vi "[P] Upload To Server.vi"() -> ()   [LabVIEW 2014]
uses:
  Sensor Reading.ctl
  Enum.ServerUploadState.ctl
  <vilib>/regexp/Match Regular Expression.xnode
panel:
  in  "Timeout":u16
  in  "Control Port":u16
  in  "Fail Silently?":bool
  in  "Data Port":u16
  in  "Server Address":string
  in  "Message Q":refnum<queue>
  in  "Data Q":refnum<queue>
  in  "Sensor Reading":T1
  # "INPUT PARAMETERS"
  # "INTERNAL VARIABLES - could possibly be set programatically..."
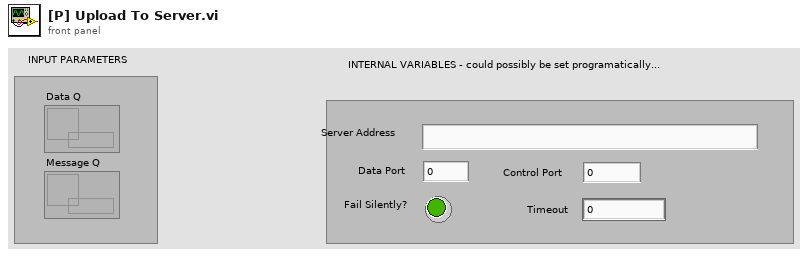
[diagram p1: front panel]
types:
  T1 = typedef "Sensor Reading.ctl" = cluster{"Sensor Name":string, "Timestamp":string, "Data Chunk":string}
  T2 = enum16{"Standard", "Buffered", "CRLF", "Immediate"}
  T3 = typedef "Enum.ServerUploadState.ctl" = enum16{"NotConnected", "Connected", "Error"}
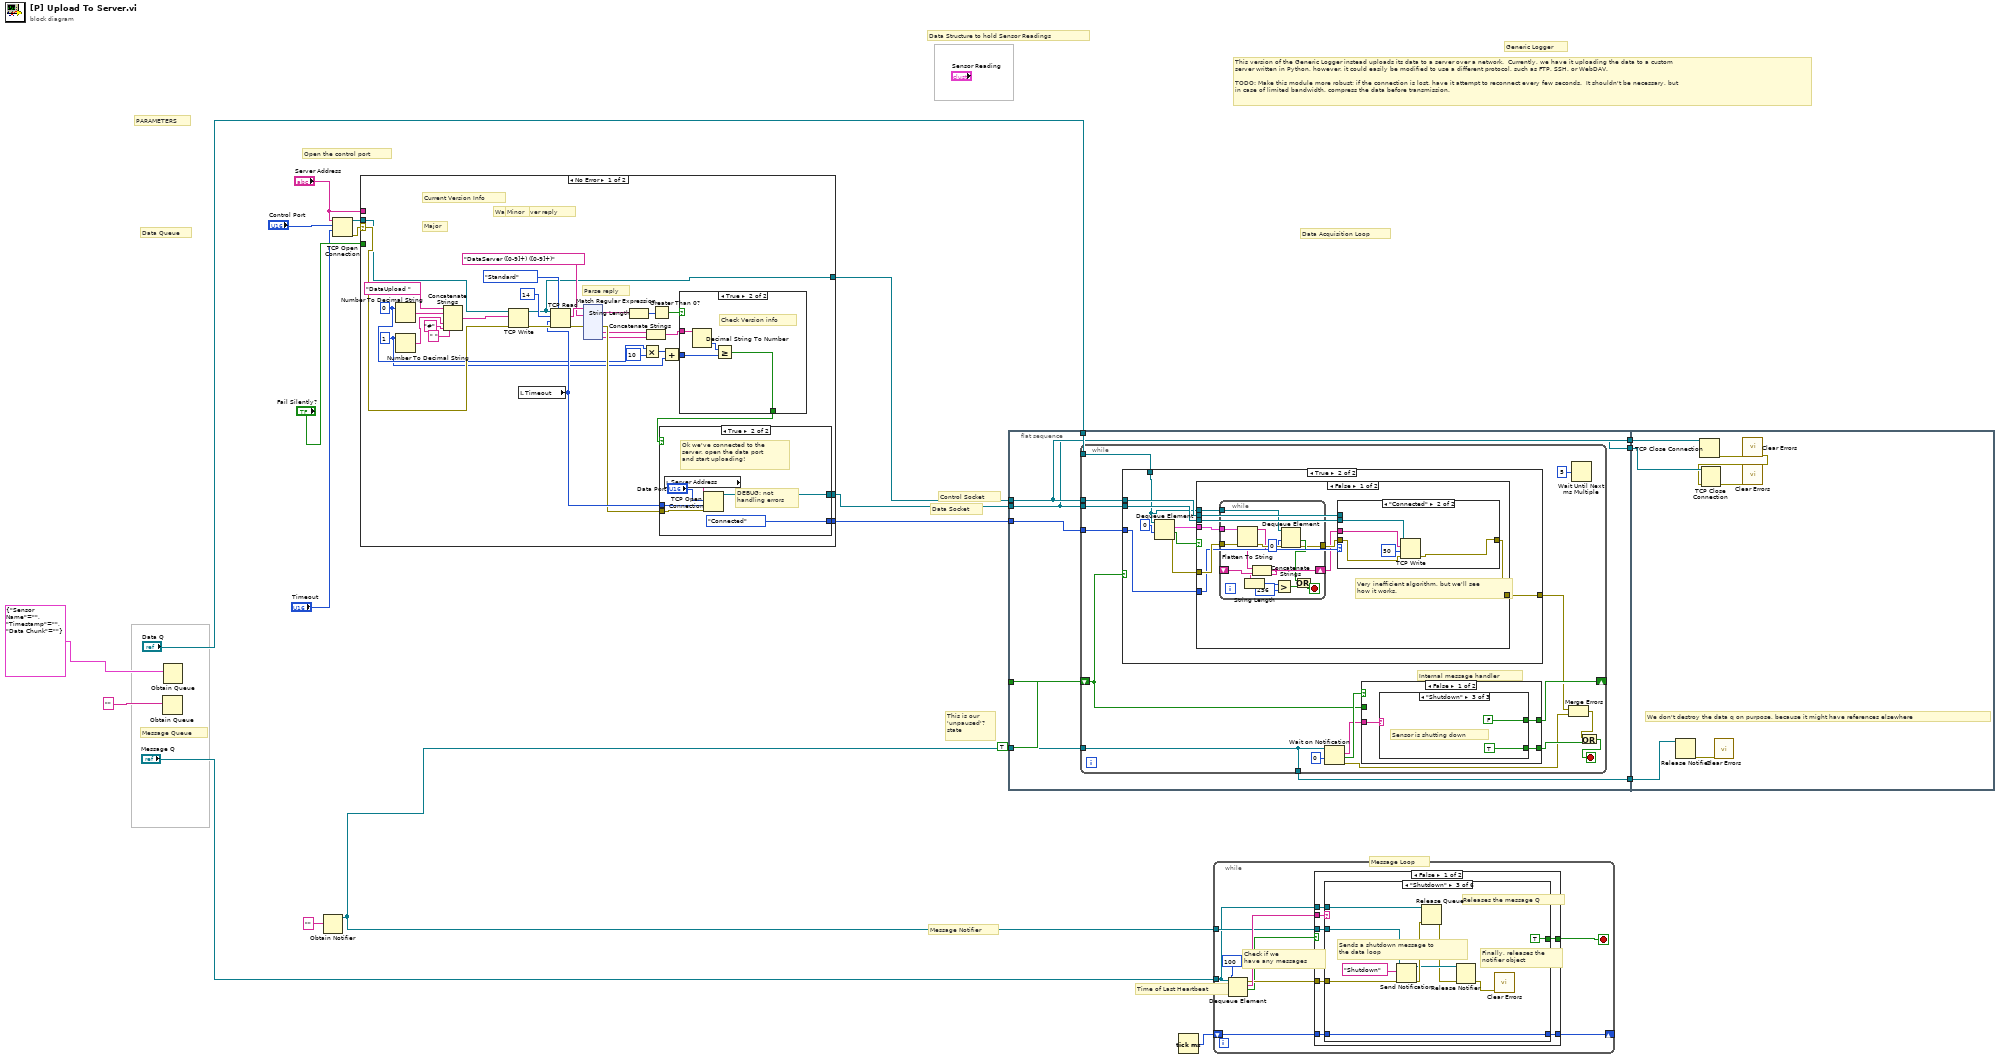
[diagram p0: block diagram]
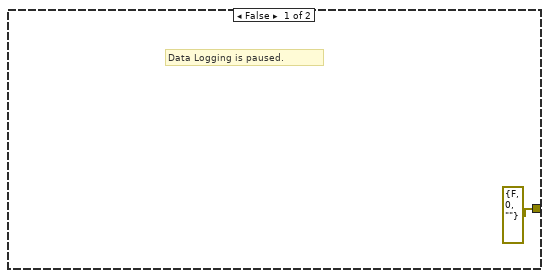
[diagram p2: hidden frame]
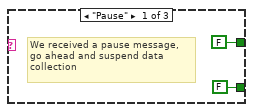
[diagram p5: hidden frame]
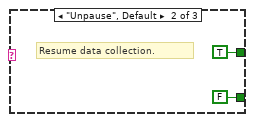
[diagram p6: hidden frame]
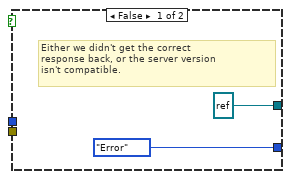
[diagram p8: hidden frame]
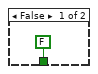
[diagram p9: hidden frame]
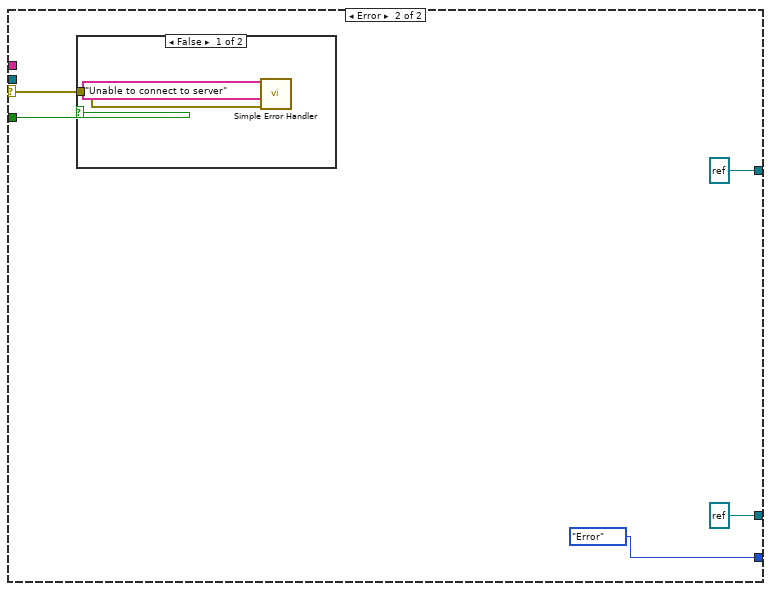
[diagram p10: hidden frame]
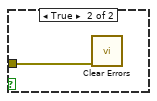
[diagram p11: hidden frame]
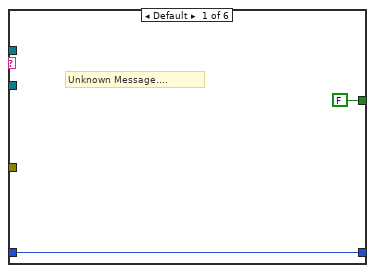
[diagram p12: hidden frame]
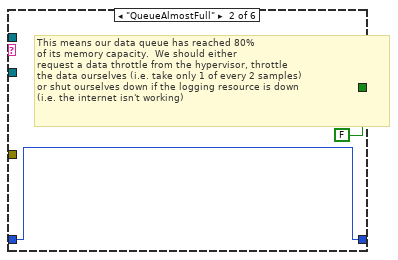
[diagram p13: hidden frame]
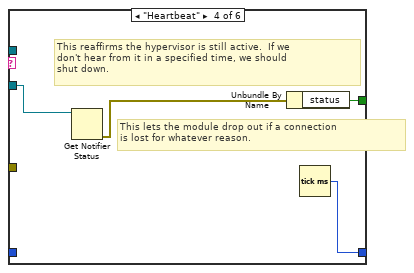
[diagram p14: hidden frame]
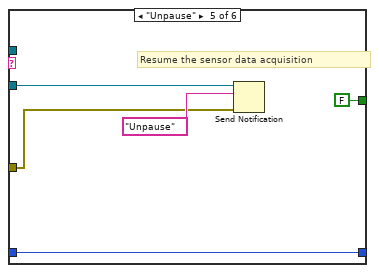
[diagram p15: hidden frame]
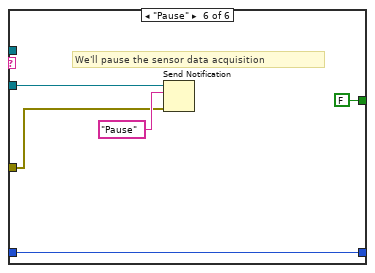
[diagram p16: hidden frame]
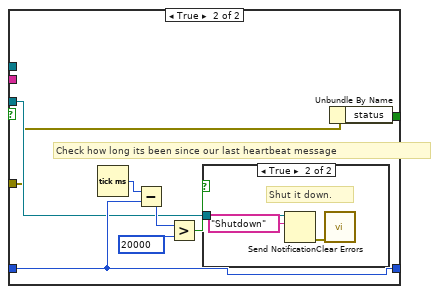
[diagram p17: hidden frame]
diagram:
  # "Control Socket"
  # "Data Socket"
  # "Open the control port"
  # "Data Acquisition Loop"
  # "Time of Last Heartbeat"
  # "This version of the Generic Logger instead uploads its data to a server over a network.  Currently, we have it uploading the data to a custom\nserver written in Python, however, it could easily be modified to use a different protocol, such as FTP, SSH, or WebDAV.\n\nTODO: Make this module more robust; if the connection is lost, have it attempt to reconnect every few seconds.  It shouldn't be necessary, but \nin case of limited bandwidth, compress the data before transmission."
  # "This is our\n'unpaused'?\nstate"
  # "Data Structure to hold Sensor Readings"
  # "Message Loop"
  # "Message Notifier"
  # "Message Queue"
  # "Data Queue"
  # "PARAMETERS"
  # "Generic Logger"
  n1 = Obtain Queue(element data type="" ("element")) -> ()  [unwired: 4 in, 3 out]
  n2 = Obtain Queue(element data type=T1 {"Sensor Name"="", "Timestamp"="", "Data Chunk"=""} ("element")) -> ()  [unwired: 4 in, 3 out]
  n3 = Obtain Notifier(notification data type="") -> (notifier out=w20:refnum<notifier>)  [unwired: 3 in, 2 out]
  n4 = TCP Open Connection(address="Server Address", remote port or service name="Control Port", timeout ms (60000)="Timeout") -> (connection ID=w11:refnum<k5>, error out=w13:errorcluster)  [unwired: 2 in]
  n5 = case shown="No Error" w13 {
    selector: w13 -> [w51 w185]
    tunnel: [w33 refnum<k5> refnum ("connection ID")] -> w16
    tunnel: "Server Address" -> [_ _]
    tunnel: "Fail Silently?" -> [_ w186]
    tunnel: w11 -> [w50 _]
    tunnel: [w34 Enum.ServerUploadState."Error" ("UploadState")] -> w9
    tunnel: [w32 refnum<k5> refnum ("connection ID")] -> w8
    frame No Error {
      w25 = 1
      w28 = 0
      # "Parse reply"
      # "Wait for server reply"
      # "Minor"
      # "Major"
      # "Current Version Info"
      n6 = Number To Decimal String(number=w28) -> (decimal integer string=w39:string)  [unwired: 1 in]
      n7 = Number To Decimal String(number=w25) -> (decimal integer string=w22:string)  [unwired: 1 in]
      n8 = Concatenate Strings("DataUpload " ("data in"), w39, " " ("string"), w22, "#" ("string")) -> (w38:string)
      n9 = TCP Write(connection ID=w50, data in=w38, error in (no error)=w51) -> (connection ID out=w33:refnum<k5>, error out=w44:errorcluster)  [unwired: 1 in, 1 out]
      n10 = local read "Timeout"() -> (w36:u16)
      n11 = TCP Read(connection ID=w33, bytes to read=14, error in (no error)=w44, 7:T2."Standard" ("mode (standard)"), 9:w36) -> (data out=w47:string, error out=w45:errorcluster)  [unwired: 1 out]
      n12 = xnode "Match Regular Expression"("input string"=w47, "regular expression"="DataServer ([0-9]+) ([0-9]+)", "error in"=w45) -> ("whole match"=w43:string, "error out"=w35:errorcluster, "submatch 1"=w31:string, "submatch 2"=w30:string)  [unwired: 3 in, 3 out]
      n13 = String Length(string=w43) -> (length=w42:i32)
      n14 = Multiply(x=w28, y=10) -> (x*y=w26:i32)
      n15 = Concatenate Strings(w31, w30) -> (w29:string)
      n16 = Greater Than 0?(x=w42) -> (x > 0?=w41:bool)
      n17 = Add(x=w26, y=w25) -> (x+y=w24:i32)
      n18 = case shown="True" w41 {
        tunnel: [FALSE w61] -> w37
        tunnel: w29 -> [_ w63]
        tunnel: w24 -> [_ w62]
        frame False {
        }
        frame True {
          # "Check Version info"
          n19 = Decimal String To Number(string=w63) -> (number=w64:i32)  [unwired: 2 in, 1 out]
          n20 = Greater Or Equal?(x=w64, y=w62) -> (x >= y?=w61:bool)
        }
      }
      n21 = case shown="True" w37 {
        tunnel: w36 -> [_ w57]
        tunnel: w35 -> [_ w56]
        tunnel: [Enum.ServerUploadState."Error" ("UploadState") Enum.ServerUploadState."Connected" ("UploadState")] -> w34
        tunnel: [refnum<k5> refnum ("connection ID") w54] -> w32
        frame False {
          # "Either we didn't get the correct\nresponse back, or the server version\nisn't compatible."
        }
        frame True {
          # "DEBUG: not\nhandling errors"
          # "Ok we've connected to the\nserver, open the data port\nand start uploading!"
          n22 = local read "Server Address"() -> (w58:string)
          n23 = TCP Open Connection(address=w58, remote port or service name="Data Port", timeout ms (60000)=w57, error in (no error)=w56) -> (connection ID=w54:refnum<k5>)  [unwired: 1 in, 1 out]
        }
      }
    }
    frame Error {
      n24 = case shown="False" w186 {
        tunnel: w185 -> [w188 w189]
        frame False {
          n25 = call <vilib>:"Simple Error Handler.vi"("error source (\" \")"="Unable to connect to server" ("error source (\" \")"), "error in (no error)"=w188) -> ()  [unwired: 3 in, 5 out]
        }
        frame True {
          n26 = call <vilib>:"Clear Errors.vi"("error in (no error)"=w189) -> ()  [unwired: 5 in, 2 out]
        }
      }
    }
  }
  n27 = flat-sequence {
    tunnel: w20 -> [w196]
    tunnel: TRUE -> [w195]
    tunnel: w16 -> [w192]
    tunnel: w9 -> [w194]
    tunnel: w8 -> [w191]
    tunnel: "Data Q" -> [w193]
    tunnel: [w192] -> w3
    tunnel: [w191] -> w2
    tunnel: [w190] -> w1
    tunnel: w3 -> [w269]
    tunnel: w2 -> [w268]
    tunnel: w1 -> [w264]
    frame #0 {
      n28 = while {
        tunnel: w193 -> [w204]
        tunnel: w196 -> [w197]
        shift-right: [w209] -> _
        shift-left: w195 -> [w208]
        tunnel: w192 -> [w200]
        tunnel: w194 -> [w199]
        tunnel: w191 -> [w198]
        tunnel: [w197] -> w190
        stop <- w206 stop-if-true
        # "Internal message handler"
        n29 = case shown="True" w208 {
          tunnel: w204 -> [_ w214]
          tunnel: [errorcluster {"status"=FALSE, "code"=0, "source"=""} ("error out") w219] -> w203
          tunnel: w200 -> [_ w217]
          tunnel: w199 -> [_ w216]
          tunnel: w198 -> [_ w215]
          frame False {
            # "Data Logging is paused."
          }
          frame True {
            n30 = Dequeue Element(queue=w214, timeout in ms (-1)=0) -> (element=w220:T1, timed out?=w221:bool, error out=w218:errorcluster)  [unwired: 1 in, 1 out]
            n31 = case shown="False" w221 {
              tunnel: w220 -> [w231 _]
              tunnel: [w229 w252] -> w219
              tunnel: w218 -> [w230 w252]
              tunnel: w217 -> [w227 _]
              tunnel: w216 -> [w228 _]
              tunnel: w215 -> [w226 _]
              tunnel: w214 -> [w225 _]
              frame False {
                # "Very inefficient algorithm, but we'll see\nhow it works."
                # "UPLOAD HERE"
                n32 = while {
                  tunnel: w231 -> [w245]
                  tunnel: w225 -> [w242]
                  shift-right: [w238] -> w223
                  shift-left: _ -> [w240]
                  tunnel: w230 -> [w244]
                  tunnel: [w232] -> w224
                  stop <- w233 stop-if-true
                  n33 = Flatten To String(anything=w245, error in (no error)=w244) -> (data string=w239:string, error out=w243:errorcluster)  [unwired: 2 in, 1 out]
                  n34 = Concatenate Strings(w239, w240) -> (w238:string)
                  n35 = String Length(string=w238) -> (length=w237:i32)
                  n36 = Greater?(x=w237, y=256) -> (0:w234:bool)
                  n37 = Dequeue Element(queue=w242, timeout in ms (-1)=0, error in (no error)=w243) -> (timed out?=w235:bool, error out=w232:errorcluster)  [unwired: 2 out]
                  n38 = Or(x=w235, y=w234) -> (x .or. y?=w233:bool)
                }
                n39 = case shown="\"Connected\"" w228 {
                  tunnel: w224 -> [w246 w251]
                  tunnel: [w246 w247] -> w229
                  tunnel: w227 -> [_ _]
                  tunnel: w226 -> [_ w249]
                  tunnel: w223 -> [_ w248]
                  frame "NotConnected", Default {
                  }
                  frame "Connected" {
                    n40 = TCP Write(connection ID=w249, data in=w248, error in (no error)=w251, 9:50 ("timeout ms (25000)")) -> (error out=w247:errorcluster)  [unwired: 2 out]
                  }
                }
              }
              frame True {
              }
            }
          }
        }
        n41 = Wait on Notification(notifier=w197, timeout in ms (-1)=0) -> (notification=w210:string, timed out?=w211:bool, error out=w202:errorcluster)  [unwired: 2 in, 1 out]
        n42 = case shown="False" w211 {
          tunnel: w210 -> [w255 _]
          tunnel: [w254 _] -> w207
          tunnel: [w253 w262] -> w209
          tunnel: w208 -> [_ w262]
          frame False {
            n43 = case shown="\"Shutdown\"" w255 {
              tunnel: [FALSE FALSE TRUE] -> w254
              tunnel: [FALSE TRUE FALSE] -> w253
              frame "Pause" {
                # "We received a pause message,\ngo ahead and suspend data collection"
              }
              frame "Unpause", Default {
                # "Resume data collection."
              }
              frame "Shutdown" {
                # "Sensor is shutting down"
              }
            }
          }
          frame True {
          }
        }
        n44 = Merge Errors(w203, w202) -> (w201:errorcluster)
        n45 = Wait Until Next ms Multiple(millisecond multiple=u32 5) -> ()  [unwired: 1 out]
        n46 = Or(x=w201, y=w207) -> (x .or. y?=w206:bool)
      }
    }
    frame #1 {
      # "We don't destroy the data q on purpose, because it might have references elsewhere"
      n47 = Release Notifier(notifier=w264) -> (error out=w263:errorcluster)  [unwired: 2 in, 2 out]
      n48 = TCP Close Connection(connection ID=w269) -> (error out=w267:errorcluster)  [unwired: 2 in, 1 out]
      n49 = call <vilib>:"Clear Errors.vi"("error in (no error)"=w263) -> ()  [unwired: 5 in, 2 out]
      n50 = call <vilib>:"Clear Errors.vi"("error in (no error)"=w267) -> ("error out"=w266:errorcluster)  [unwired: 5 in, 1 out]
      n51 = TCP Close Connection(connection ID=w268, error in (no error)=w266) -> (error out=w265:errorcluster)  [unwired: 1 in, 1 out]
      n52 = call <vilib>:"Clear Errors.vi"("error in (no error)"=w265) -> ()  [unwired: 5 in, 2 out]
    }
  }
  n53 = Tick Count (ms)() -> (millisecond timer value=w17:u32)
  n54 = while {
    tunnel: "Message Q" -> [w275]
    tunnel: w20 -> [w276]
    shift-right: [w270] -> _
    shift-left: w17 -> [w271]
    stop <- w277 stop-if-true
    # "Check if we \nhave any messages"
    n55 = Dequeue Element(queue=w275, timeout in ms (-1)=100) -> (element=w278:string, timed out?=w272:bool, error out=w274:errorcluster)  [unwired: 1 in, 1 out]
    n56 = case shown="False" w272 {
      tunnel: w278 -> [w279 _]
      tunnel: [w285 w314] -> w277
      tunnel: w276 -> [w284 w317]
      tunnel: w275 -> [w283 _]
      tunnel: w274 -> [w282 w315]
      tunnel: w271 -> [w281 w318]
      tunnel: [w280 w318] -> w270
      frame False {
        n57 = case shown="\"Shutdown\"" w279 {
          tunnel: [FALSE FALSE TRUE w300 FALSE FALSE] -> w285
          tunnel: w284 -> [_ _ w297 w302 w306 w310]
          tunnel: w283 -> [_ _ w298 _ _ _]
          tunnel: w282 -> [_ _ w296 _ w307 w311]
          tunnel: w281 -> [w286 w288 w291 _ w304 w309]
          tunnel: [w286 w288 w291 w303 w304 w309] -> w280
          frame Default {
            # "Unknown Message...."
          }
          frame "QueueAlmostFull" {
            # "This means our data queue has reached 80%\nof its memory capacity.  We should either\nrequest a data throttle from the hypervisor, throttle\nthe data ourselves (i.e. take only 1 of every 2 samples)\nor shut ourselves down if the logging resource is down\n(i.e. the internet isn't working)"
          }
          frame "Shutdown" {
            # "Finally, releases the\nnotifier object"
            # "Releases the message Q"
            # "Sends a shutdown message to \nthe data loop"
            n58 = Send Notification(notification="Shutdown", notifier=w297, error in (no error)=w296) -> (notifier out=w293:refnum<notifier>, error out=w295:errorcluster)
            n59 = Release Queue(queue=w298, error in (no error)=w295) -> (error out=w292:errorcluster)  [unwired: 1 in, 2 out]
            n60 = Release Notifier(notifier=w293, error in (no error)=w292) -> (error out=w290:errorcluster)  [unwired: 1 in, 2 out]
            n61 = call <vilib>:"Clear Errors.vi"("error in (no error)"=w290) -> ()  [unwired: 5 in, 2 out]
          }
          frame "Heartbeat" {
            # "This lets the module drop out if a connection\nis lost for whatever reason."
            # "This reaffirms the hypervisor is still active.  If we\ndon't hear from it in a specified time, we should\nshut down."
            n62 = Get Notifier Status(notifier=w302) -> (error out=w301:errorcluster)  [unwired: 1 in, 4 out]
            n63 = Unbundle By Name(w301) -> ("status"=w300:bool)
            n64 = Tick Count (ms)() -> (millisecond timer value=w303:u32)
          }
          frame "Unpause" {
            # "Resume the sensor data acquisition"
            n65 = Send Notification(notification="Unpause", notifier=w306, error in (no error)=w307) -> ()  [unwired: 2 out]
          }
          frame "Pause" {
            # "We'll pause the sensor data acquisition"
            n66 = Send Notification(notification="Pause", notifier=w310, error in (no error)=w311) -> ()  [unwired: 2 out]
          }
        }
      }
      frame True {
        # "DEBUG: set to 20 sec"
        # "Check how long its been since our last heartbeat message"
        # "Do any maintenance we might\nneed to do.  Sensor still active?\nResources still valid? etc"
        # "We've not received a message in 100 ms...."
        n67 = Tick Count (ms)() -> (millisecond timer value=w321:u32)
        n68 = Subtract(x=w321, y=w318) -> (x-y=w320:u32)
        n69 = Greater?(x=w320, y=u32 20000) -> (0:w316:bool)
        n70 = case shown="True" w316 {
          tunnel: w317 -> [_ w324]
          frame False {
          }
          frame True {
            # "Shut it down."
            n71 = Send Notification(notification="Shutdown", notifier=w324) -> (error out=w322:errorcluster)  [unwired: 1 in, 1 out]
            n72 = call <vilib>:"Clear Errors.vi"("error in (no error)"=w322) -> ()  [unwired: 5 in, 2 out]
          }
        }
        n73 = Unbundle By Name(w315) -> ("status"=w314:bool)
      }
    }
  }
